vi "Set Bitfile Path.vi"(8 "error in (no error)":errorcluster, 9 "Bitfile Path in":path, 10 "RIO Device Address in":string, 11 "Item Ref in":T1 format="%.0x") -> (0 "error out":errorcluster, 3 "Item Ref out":T1 format="%.0x")   [LabVIEW 2015, in "Engine Simulation Toolkit System Explorer.lvlib"]
uses:
  Engine Simulation Toolkit System Explorer.lvlib
  <vilib>/NI Veristand/Custom Device API/Custom Device Item Ref.ctl
  <vilib>/NI Veristand/Custom Device API/Dependent File Optional Info.ctl
  <vilib>/NI Veristand/Custom Device API/Set Item Property (Dependent File).vi
  <vilib>/NI Veristand/Custom Device API/Custom Device API.lvlib
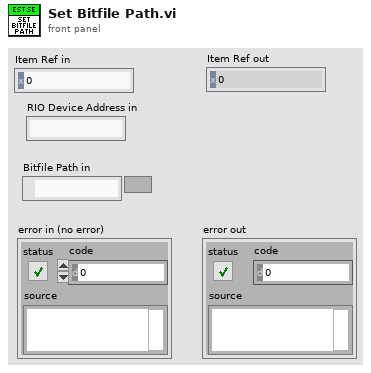
[diagram p1: front panel]
types:
  T1 = typedef "Custom Device API.lvlib/Custom Device Item Ref.ctl" = u64
  T2 = typedef "Custom Device API.lvlib/Dependent File Optional Info.ctl" = cluster{"Version":string, "RTDestination":path, "ForceDownload":bool, "SupportedTarget":string, "MD5":string}
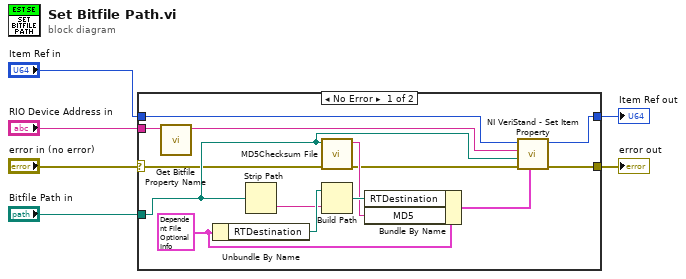
[diagram p0: block diagram]
diagram:
  n1 = case shown="No Error" "error in (no error)" {
    selector: "error in (no error)" -> [w16 w22]
    tunnel: "Bitfile Path in" -> [w20 _]
    tunnel: "RIO Device Address in" -> [w18 _]
    tunnel: "Item Ref in" -> [w17 w21]
    tunnel: [w15 w22] -> w2
    tunnel: [w7 w21] -> w1
    frame No Error {
      w13 = T2 {"Version"="1.0", "RTDestination"=path "c:/ni-rt/NIVeriStand/Custom Devices/Engine Simulation Toolkit", "ForceDownload"=FALSE, "SupportedTarget"="All", "MD5"=""} ("OptionalInfo")
      n2 = call "Get Bitfile Property Name.vi"("RIO Device Address in"=w18) -> ("Bitfile Property Name"=w19:string)  [unwired: 10 in]
      n3 = Unbundle By Name(w13) -> ("RTDestination"=w12:path)
      n4 = Strip Path(path=w20) -> (name=w11:string)  [unwired: 1 out]
      n5 = call <vilib>:"MD5Checksum File.vi"("error in (no error)"=w16, "Path"=w20) -> ("error out"=w8:errorcluster, "MD5 message-digest"=w9:string)  [unwired: 8 in]
      n6 = Build Path(base path=w12, name or relative path=w11) -> (appended path=w10:path)
      n7 = Bundle By Name(cluster=w13, "RTDestination"=w10, "MD5"=w9) -> (w14:T2)
      n8 = call-poly <vilib>:"NI VeriStand - Set Item Property.vi"("OptionalInfo"=w14, "error in (no error)"=w8, "Path"=w20, "Property Name"=w19, "Item Ref in"=w17) -> ("error out"=w15:errorcluster, "Item Ref out"=w7:T1)  [unwired: 4 in, 1 out]
    }
    frame Error {
    }
  }
  "error out" <- w2
  "Item Ref out" <- w1
